vi "Run Bfr Rx - Prepend Size.vi"(8 "error in (no error)":errorcluster, 10 "Data in":u8[](array[numeric]), 11 "Data Buffer in":u64 format="%016x") -> (0 "error out":errorcluster, 2 "Data out":u8[](array[numeric]), 3 "Data Buffer out":u64 format="%016x")   [LabVIEW 2016, in "UDP-Custom-Device Engine.lvlib"]
uses:
  UDP-Custom-Device Engine.lvlib
  <vilib>/NI Veristand/VeriStand Data/Library/Pointer Operations/Pointer.Write (I32).vi
  <vilib>/NI Veristand/VeriStand Data/Library/VeriStand Data.lvlib
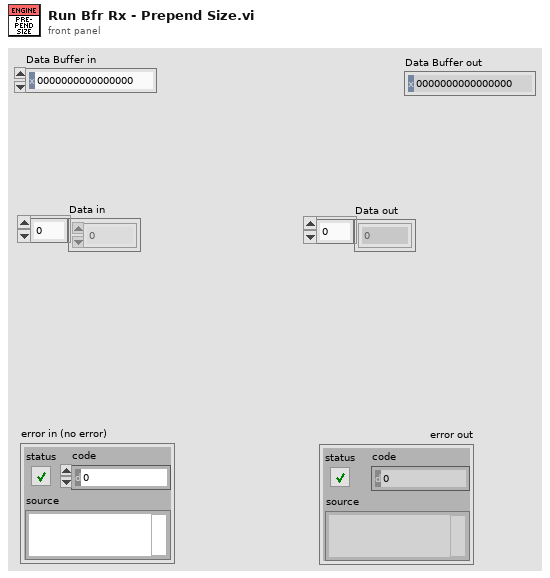
[diagram p1: front panel]
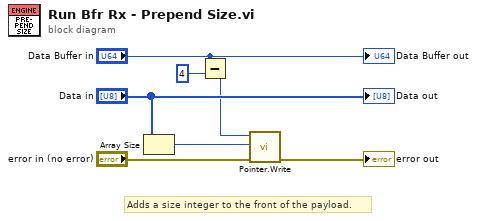
[diagram p0: block diagram]
diagram:
  # "Adds a size integer to the front of the payload."
  n1 = Array Size(array="Data in") -> (size(s)=w1:i32)
  n2 = Subtract(x="Data Buffer in", y=u64 4) -> (x-y=w2:u64)
  n3 = call-poly <vilib>:"Pointer.Write.vi"("error in (no error)"="error in (no error)", "value"=w1, "pointer in"=w2) -> ("error out"=→"error out":errorcluster)  [unwired: 6 in, 2 out]
  "Data out" <- "Data in"
  "Data Buffer out" <- "Data Buffer in"
